vi "Mass Dispense Control (SubVI).vi"(0 "Weight (Grams)":dbl, 1 "Dispense Setpoint (%)":dbl=2.0, 2 "Fill Setpoint (g)":dbl=1000.0, 3 "Settings":T2={"ON Settings"={"Enable Dynamic Setpoint?"=TRUE, "Enable Dynamic Dispense Time?"=TRUE, "Enable Drain Rate Functions"=TRUE, "Dispense Sample Time (s)"=0.5, "Dispense Slope Ave"=0, "ON Timeout (sec)"=600.0, "1st Setpoint (% of Target)"=0.0, "2nd Setpoint (% of Target)"=0.0, "3rd Setpoint (% of Target)"=0.0, "Measure Dispense Delay (sec)"=0.0, "Settle Slope Sample Time (s)"=0.0}, "OFF Settings"={"Drain Sample Time (s)"=0.5, "Drain Rate Ave Size"=5, "Drain Rate Limits (± g/sec)"=10.0, "Level Slope Range (± g/sec)"=0.25, "OFF Timeout (sec)"=0.0, "Near SP Slope Level (± g/sec)"=0.01, "Near Setpoint Threshold (%)"=95.0}, "Overshoot Settings"={"Time Limit (s)"=60.0, "Container MAX (g)"=1500.0, "Max FILL Slope (+/- g/sec)"=10.0, "% Overshot to Enable (>)"=0.25}, "FILL Timeout (s)"=300.0, "Full Settle Time (s)"=20.0, "Pre-Hydrate \nSpray Time (s)"=10.0, "Pre-Hydrate \nWait Time (s)"=30.0}, 4 "Product Weight (g)":dbl, 5 "Overshoot Adjust?":bool=TRUE, 6 "STOP Dispense":bool, 8 "START Dispense":bool) -> (14 "Signals":T4, 16 "Values":T5 {"Drain Time (s)" format="%.2f"; "Drain Rate (g/sec)" format="%.2f"; "Time Elapsed (s)" format="%.2f"; "Time Target (s)" format="%.2f"; "Dynamic Setpoint (g)" format="%.2f"; "Static Setpoint (g)" format="%.2f"; "Grams to Setpoint" format="%.2f"; "Adjusted Mass (g)" format="%.2f"; "Dispense Rate (g/sec)" format="%.2f"; "Fill Mass (g)" format="%.2f"; "Fill Rate (g/sec)" format="%.2f"}, 17 "Product Values":T1, 18 "Hydration (g)":dbl, 19 "Dispense Mode":T3(ring))   [LabVIEW 2012]
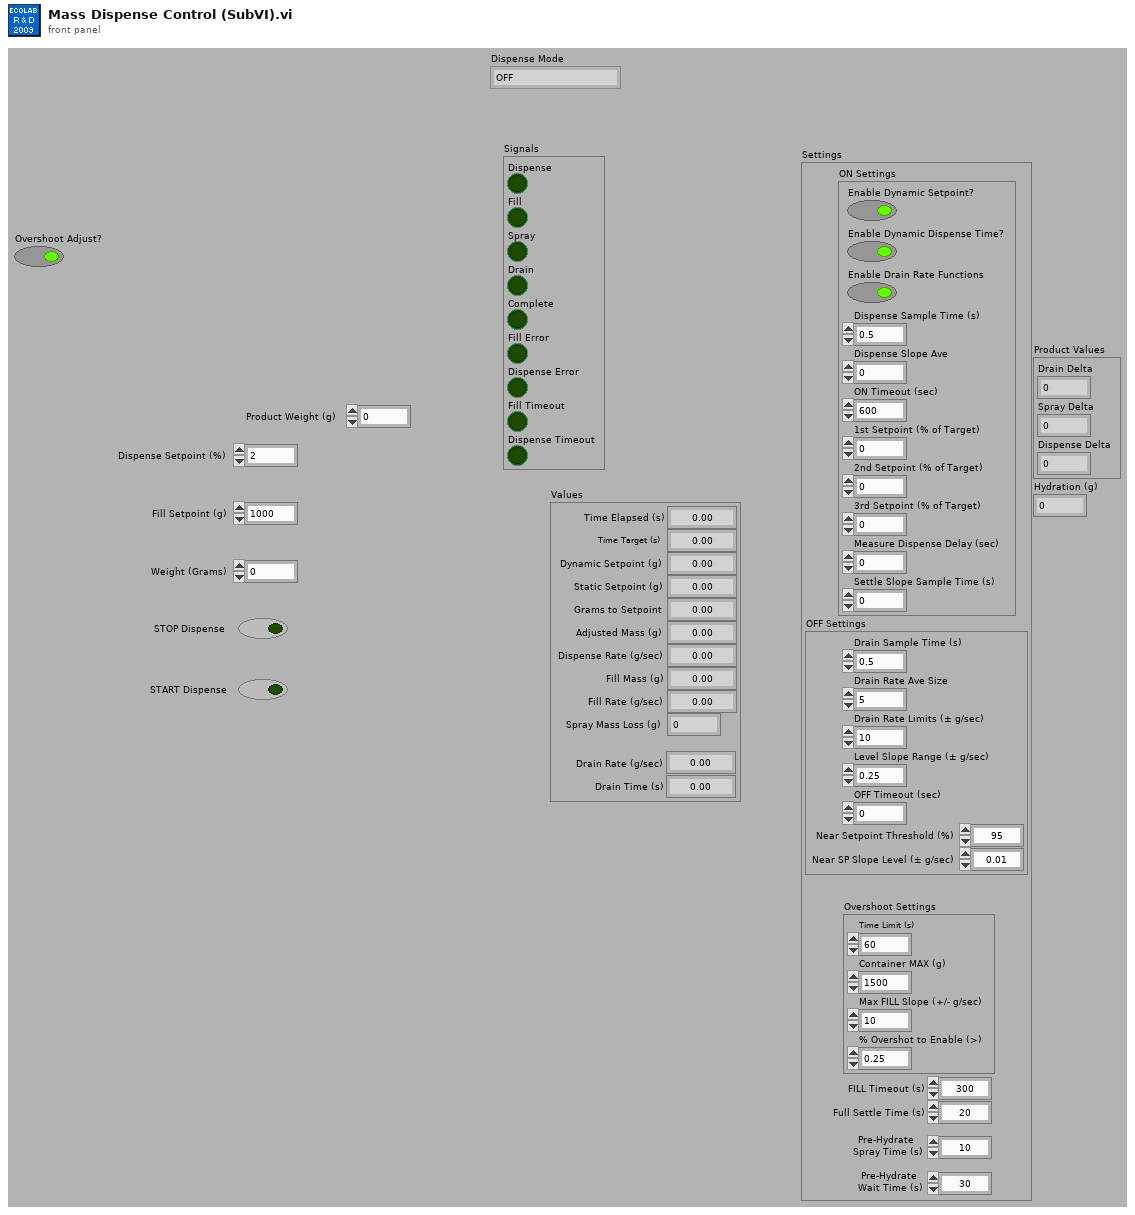
[diagram p1: front panel]
types:
  T1 = cluster{"Drain Delta":dbl, "Spray Delta":dbl, "Dispense Delta":dbl}
  T2 = cluster{"ON Settings":cluster{"Enable Dynamic Setpoint?":bool, "Enable Dynamic Dispense Time?":bool, "Enable Drain Rate Functions":bool, "Dispense Sample Time (s)":dbl, "Dispense Slope Ave":i32, "ON Timeout (sec)":dbl, "1st Setpoint (% of Target)":dbl, "2nd Setpoint (% of Target)":dbl, "3rd Setpoint (% of Target)":dbl, "Measure Dispense Delay (sec)":dbl, "Settle Slope Sample Time (s)":dbl}, "OFF Settings":cluster{"Drain Sample Time (s)":dbl, "Drain Rate Ave Size":i32, "Drain Rate Limits (± g/sec)":dbl, "Level Slope Range (± g/sec)":dbl, "OFF Timeout (sec)":dbl, "Near SP Slope Level (± g/sec)":dbl, "Near Setpoint Threshold (%)":dbl}, "Overshoot Settings":cluster{"Time Limit (s)":dbl, "Container MAX (g)":dbl, "Max FILL Slope (+/- g/sec)":dbl, "% Overshot to Enable (>)":dbl}, "FILL Timeout (s)":dbl, "Full Settle Time (s)":dbl, "Pre-Hydrate \nSpray Time (s)":dbl, "Pre-Hydrate \nWait Time (s)":dbl}
  T3 = enum16{"OFF", "INITIAL", "FILL", "DISPENSE", "ADJUST"}
  T4 = cluster{"Dispense":bool, "Fill":bool, "Spray":bool, "Drain":bool, "Complete":bool, "Fill Error":bool, "Dispense Error":bool, "Fill Timeout":bool, "Dispense Timeout":bool}
  T5 = cluster{"Time Elapsed (s)":dbl, "Time Target (s)":dbl, "Dynamic Setpoint (g)":dbl, "Static Setpoint (g)":dbl, "Grams to Setpoint":dbl, "Adjusted Mass (g)":dbl, "Dispense Rate (g/sec)":dbl, "Fill Mass (g)":dbl, "Fill Rate (g/sec)":dbl, "Spray Mass Loss (g)":dbl, "Drain Rate (g/sec)":dbl, "Drain Time (s)":dbl}
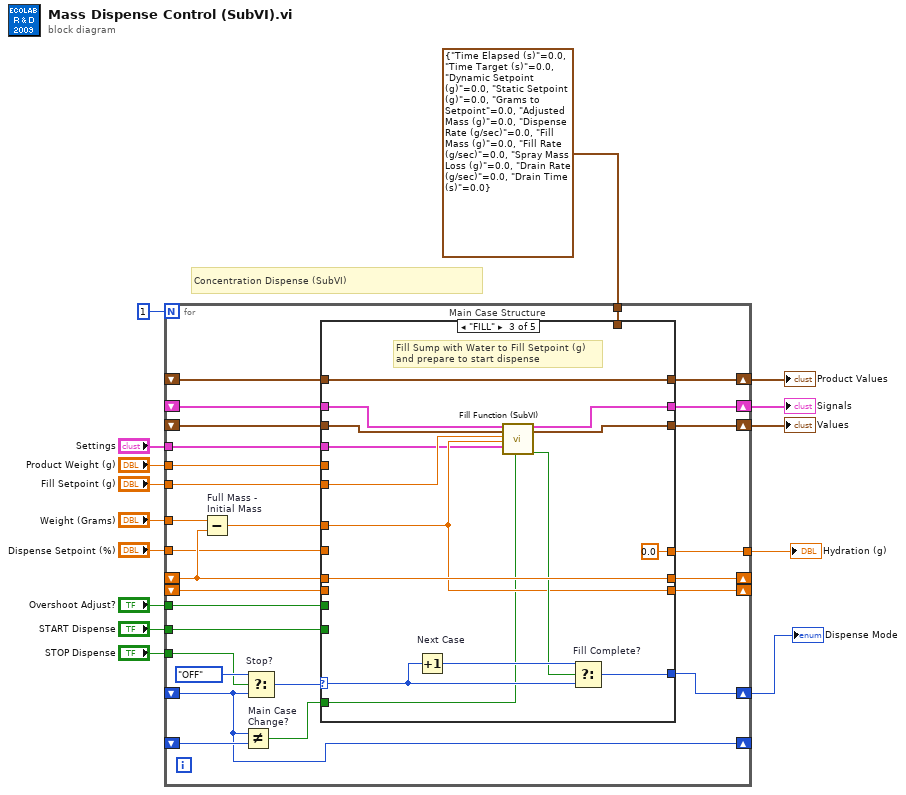
[diagram p0: block diagram]
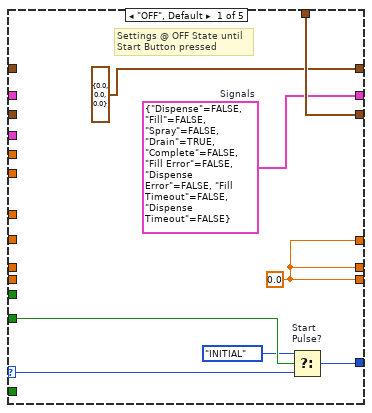
[diagram p2: hidden frame]
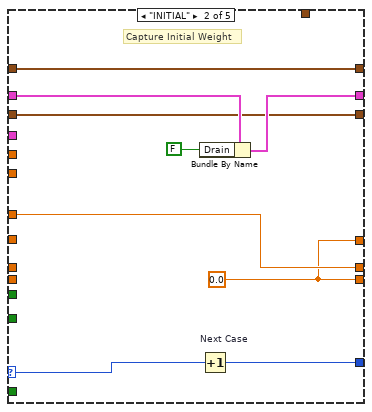
[diagram p3: hidden frame]
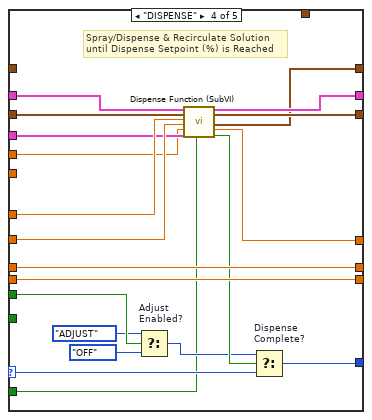
[diagram p4: hidden frame]
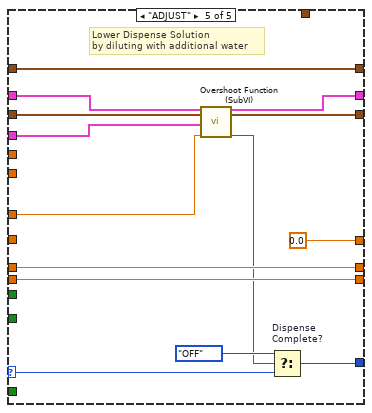
[diagram p5: hidden frame]
diagram:
  # "Concentration Dispense (SubVI)"
  n1 = for {
    N: 1 -> [_]
    tunnel: "Weight (Grams)" -> [w35]
    shift-right: [w42] -> w5
    shift-left: _ -> [w16]
    tunnel: "Fill Setpoint (g)" -> [w30]
    tunnel: "Dispense Setpoint (%)" -> [w26]
    shift-right: [w41] -> w7
    shift-left: _ -> [w31]
    shift-right: [w40] -> _
    shift-left: _ -> [w36]
    tunnel: "START Dispense" -> [w39]
    tunnel: "STOP Dispense" -> [w37]
    shift-right: [w34] -> _
    shift-left: _ -> [w33]
    tunnel: "Settings" -> [w25]
    tunnel: T5 {"Time Elapsed (s)"=0.0, "Time Target (s)"=0.0, "Dynamic Setpoint (g)"=0.0, "Static Setpoint (g)"=0.0, "Grams to Setpoint"=0.0, "Adjusted Mass (g)"=0.0, "Dispense Rate (g/sec)"=0.0, "Fill Mass (g)"=0.0, "Fill Rate (g/sec)"=0.0, "Spray Mass Loss (g)"=0.0, "Drain Rate (g/sec)"=0.0, "Drain Time (s)"=0.0} -> [w29]
    shift-right: [w28] -> w8
    shift-left: _ -> [w27]
    tunnel: "Overshoot Adjust?" -> [w24]
    tunnel: "Product Weight (g)" -> [w23]
    shift-right: [w22] -> w2
    shift-left: _ -> [w21]
    tunnel: [w20] -> w1
    shift-right: [w16] -> _
    shift-left: _ -> [w19]
    n2 = Subtract "Full Mass -\nInitial Mass"(x=w35, y=w36) -> (x-y=w32:dbl)
    n3 = Not Equal? "Main Case\nChange?"(x=w16, y=w19) -> (x != y?=w17:bool)
    n4 = Select "Stop?"(t=T3."OFF" ("Mode (Read)"), s=w37, f=w16) -> (s? t:f=w18:T3)
    n5 = case "Main Case Structure" shown="\"FILL\"" w18 {
      selector: w18 -> [w49 w59 w73 w91 w99]
      tunnel: w32 -> [_ w58 w67 w85 w97]
      tunnel: [w48 w57 w72 w94 w101] -> w42
      tunnel: w30 -> [_ _ w70 _ _]
      tunnel: [w46 w55 w66 w89 w105] -> w41
      tunnel: w31 -> [_ w56 w69 w90 w106]
      tunnel: [w43 w58 w71 w93 w108] -> w40
      tunnel: w36 -> [_ _ w71 w93 w108]
      tunnel: w39 -> [w50 _ _ _ _]
      tunnel: [w43 w51 w67 w92 w107] -> w34
      tunnel: w33 -> [_ _ _ w92 w107]
      tunnel: w29 -> [w47 _ _ _ _]
      tunnel: [w47 w53 w64 w86 w103] -> w28
      tunnel: w27 -> [_ w53 w65 w88 w104]
      tunnel: w26 -> [_ _ _ w84 _]
      tunnel: w25 -> [_ _ w61 w79 w98]
      tunnel: w24 -> [_ _ _ w83 _]
      tunnel: w23 -> [_ _ _ w78 _]
      tunnel: [T1 {"Drain Delta"=0.0, "Spray Delta"=0.0, "Dispense Delta"=0.0} ("Product Values") w52 w63 w77 w96] -> w22
      tunnel: w21 -> [_ w52 w63 _ w96]
      tunnel: [w43 w51 0.0 ("Hydration (g)") w76 0.0 ("Hydration (g)")] -> w20
      tunnel: w17 -> [_ _ w60 w75 _]
      frame "OFF", Default {
        w46 = T4 {"Dispense"=FALSE, "Fill"=FALSE, "Spray"=FALSE, "Drain"=TRUE, "Complete"=FALSE, "Fill Error"=FALSE, "Dispense Error"=FALSE, "Fill Timeout"=FALSE, "Dispense Timeout"=FALSE}  # Signals
        w43 = 0.0 ("Weight (Grams)")
        # "Settings @ OFF State until\nStart Button pressed"
        n6 = Select "Start\nPulse?"(t=T3."INITIAL" ("Mode (Read)"), s=w50, f=w49) -> (s? t:f=w48:T3)
      }
      frame "INITIAL" {
        w51 = 0.0 ("Weight (Grams)")
        # "Capture Initial Weight"
        n7 = Bundle By Name(cluster=w56, "Drain"=FALSE) -> (w55:T4)
        n8 = Increment "Next Case"(x=w59) -> (x+1=w57:T3)
      }
      frame "FILL" {
        # "Fill Sump with Water to Fill Setpoint (g)\nand prepare to start dispense"
        n9 = Increment "Next Case"(x=w73) -> (x+1=w74:T3)
        n10 = call "Fill Function (SubVI).vi"("Signals IN"=w69, "Values IN"=w65, "FILL Setpoint (g)"=w70, "Measured Mass (g)"=w67, "Settings"=w61, "Main Case Change?"=w60) -> ("Signals OUT"=w66:T4, "Values OUT"=w64:T5, "Fill FN Complete"=w68:bool)  [unwired: 1 in, 10 out]
        n11 = Select "Fill Complete?"(t=w74, s=w68, f=w73) -> (s? t:f=w72:T3)
      }
      frame "DISPENSE" {
        # "Spray/Dispense & Recirculate Solution\nuntil Dispense Setpoint (%) is Reached"
        n12 = Select "Adjust\nEnabled?"(t=T3."ADJUST" ("Mode (Read)"), s=w83, f=T3."OFF" ("Mode (Read)")) -> (s? t:f=w80:T3)
        n13 = call "Dispense Function (SubVI).vi"("Signals IN"=w90, "Values IN"=w88, "Measured Mass (g)"=w85, "Main Concentration Setpoint (%)"=w84, "Product Weight (g)"=w78, "Settings"=w79, "Main Case Change?"=w75) -> ("Signals OUT"=w89:T4, "Values OUT"=w86:T5, "Product Values"=w77:T1, "Hydration (g)"=w76:dbl, "Dispense Complete?"=w87:bool)  [unwired: 8 out]
        n14 = Select "Dispense\nComplete?"(t=w80, s=w87, f=w91) -> (s? t:f=w94:T3)
      }
      frame "ADJUST" {
        # "Lower Dispense Solution\nby diluting with additional water"
        n15 = call "Overshoot Function (SubVI).vi"("Signals IN"=w106, "Values IN"=w104, "Settings"=w98, "Measured Mass (g)"=w97) -> ("Signals OUT"=w105:T4, "Values OUT"=w103:T5, "Complete"=w100:bool)  [unwired: 4 in, 9 out]
        n16 = Select "Dispense\nComplete?"(t=T3."OFF" ("Mode (Read)"), s=w100, f=w99) -> (s? t:f=w101:T3)
      }
    }
  }
  "Values" <- w8
  "Signals" <- w7
  "Dispense Mode" <- w5
  "Product Values" <- w2
  "Hydration (g)" <- w1
